vi "Read File.vi"(7 "File ID":string, 8 "error in (no error)":errorcluster, 11 "Serial Config":T2={"串口选择"="", "通讯速率"=9600, "超时时间"=200, "数据位长"=8, "奇偶校验"=enum."None", "停止位长"=10, "握手控制"=0, "字符结束"=TRUE, "结束字符"=10, "仪器地址"=1} {"结束字符" format="%.0x"; "握手控制" items=["None", "XON/XOFF", "RTS/CTS", "XON/XOFF & RTS/CTS", "DTR/DSR", "XON/XOFF & DTR/DSR"]; "停止位长" items=["1.0"=10, "1.5"=15, "2.0"=20]; "数据位长" min=5 max=8 step=1}) -> (0 "error out":errorcluster, 2 "Segment 0":T3={"Start"=enum."Non PV start", "Cycle data"=0, "Pattern link data"=0, "Tag data"="12345678"}, 3 "Segment 1 to 99":T1(array[cluster]))   [LabVIEW 2010, in "DCP551.lvlib"]
uses:
  DCP551.lvlib
  <vilib>/Instr/_visa.llb/VISA Configure Serial Port (Instr).vi
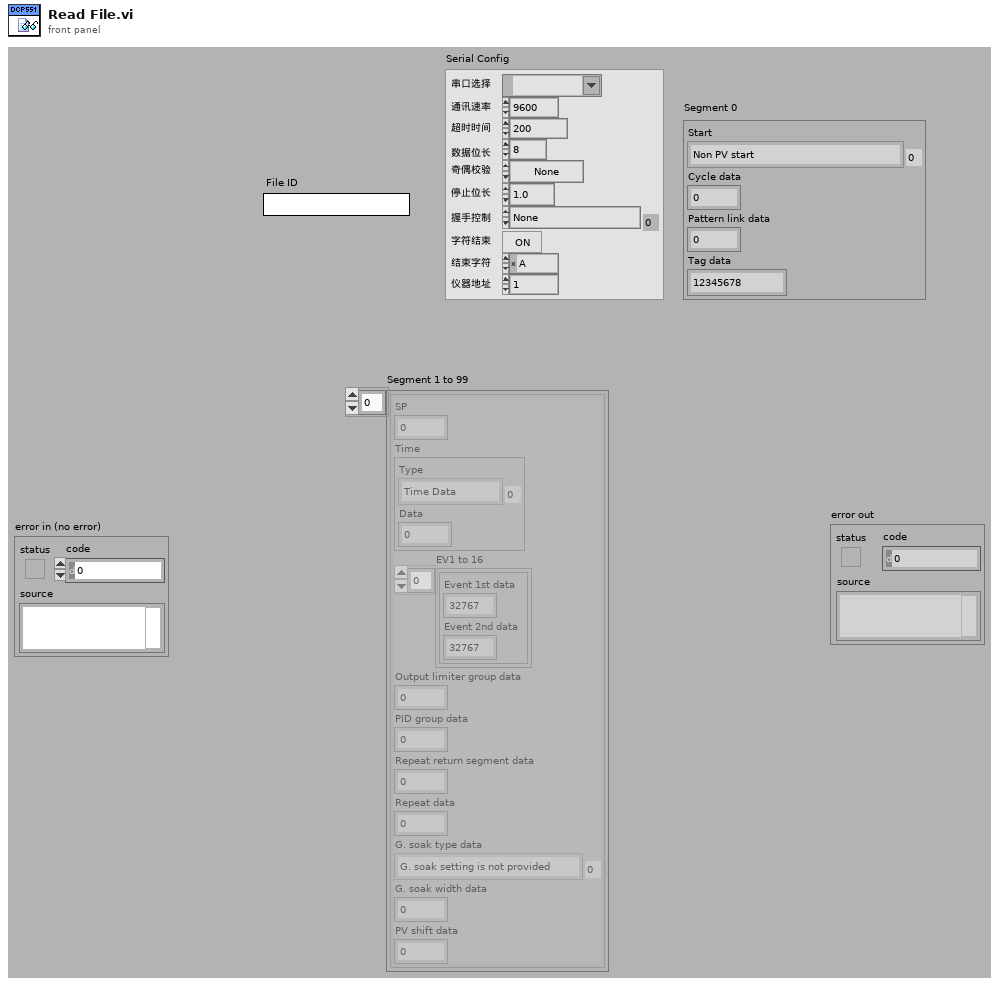
[diagram p1: front panel]
types:
  T1 = cluster{"SP":dbl, "Time":cluster{"Type":enum16{"Time Data", "delta Dtada", "SP Data"}, "Data":i32}, "EV1 to 16":cluster{"Event 1st data":i32, "Event 2nd data":i32}[], "Output limiter group data":i32, "PID group data":i32, "Repeat return segment data":i32, "Repeat data":i32, "G. soak type data":enum16{"G. soak setting is not provided", "Segment start point", "Segment end point", "Total segment"}, "G. soak width data":i32, "PV shift data":i32}[]
  T2 = cluster{"串口选择":refnum<visa-resource-name>, "通讯速率":u32, "超时时间":u32, "数据位长":u16, "奇偶校验":enum16{"None", "Odd", "Even", "Mark", "Space"}, "停止位长":u16, "握手控制":u16, "字符结束":bool, "结束字符":u8, "仪器地址":u32}
  T3 = cluster{"Start":enum16{"Non PV start", "Upward PV tart", "Downward PV start", "Either upward of downward PV start"}, "Cycle data":i32, "Pattern link data":i32, "Tag data":string}
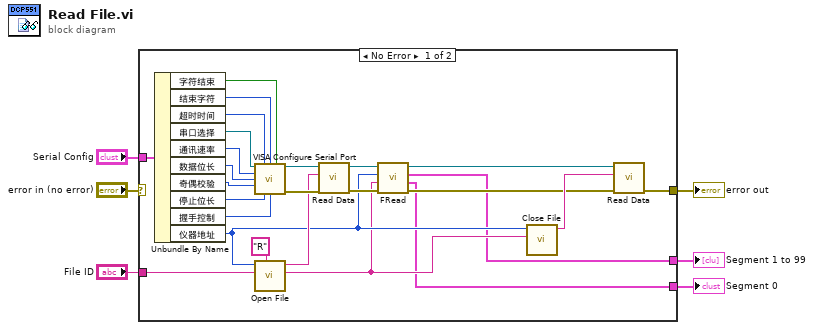
[diagram p0: block diagram]
diagram:
  n1 = case shown="No Error" "error in (no error)" {
    selector: "error in (no error)" -> [_ w31]
    tunnel: "Serial Config" -> [w21 _]
    tunnel: [w10 w31] -> w5
    tunnel: "File ID" -> [w14 _]
    tunnel: [w9 _] -> w2
    tunnel: [w7 _] -> w1
    frame No Error {
      n2 = Unbundle By Name(w21) -> ("字符结束"=w24:bool, "结束字符"=w23:u8, "超时时间"=w22:u32, "串口选择"=w30:refnum<visa-resource-name>, "通讯速率"=w29:u32, "数据位长"=w28:u16, "奇偶校验"=w27:enum16{"None", "Odd", "Even", "Mark", "Space"}, "停止位长"=w26:u16, "握手控制"=w25:u16, "仪器地址"=w15:u32)
      n3 = call-poly "VISA Configure Serial Port"("VISA resource name"=w30, "timeout (10sec)"=w22, "termination char\n(0xA = '\\n' = LF)"=w23, "Enable Termination\nChar (T)"=w24, "baud rate (9600)"=w29, "data bits (8)"=w28, "parity (0:none)"=w27, "stop bits (10: 1 bit)"=w26, "flow control (0:none)"=w25) -> ("VISA resource name out"=w20:refnum<visa-resource-name>, "error out"=w19:errorcluster)  [unwired: 1 in, 4 out]
      n4 = call "Open File.vi"("R/W"="R", "File ID"=w14, "仪器地址"=w15) -> ("OutPut"=w18:string)  [unwired: 8 in]
      n5 = call "Read Data.vi"("error in (no error)"=w19, "COMMAND"=w18, "VISA resource name in"=w20) -> ("error out"=w16:errorcluster, "VISA resource name out"=w17:refnum<visa-resource-name>)  [unwired: 6 in, 1 out]
      n6 = call "FRead.vi"("error in (no error)"=w16, "File ID"=w14, "仪器地址"=w15, "VISA resource name in"=w17) -> ("error out"=w11:errorcluster, "Segment 0"=w9:T3, "Segment 1 to 99"=w7:T1, "VISA resource name out"=w13:refnum<visa-resource-name>)  [unwired: 1 in]
      n7 = call "Close File.vi"("File ID"=w14, "仪器地址"=w15) -> ("Output"=w12:string)  [unwired: 9 in]
      n8 = call "Read Data.vi"("error in (no error)"=w11, "COMMAND"=w12, "VISA resource name in"=w13) -> ("error out"=w10:errorcluster)  [unwired: 6 in, 2 out]
    }
    frame Error {
    }
  }
  "Segment 0" <- w2
  "error out" <- w5
  "Segment 1 to 99" <- w1
